vi "XYZ Joystick.vi"(0 "LSID":i32, 7 "Joystick on?":bool, 11 "error in (no error)":errorcluster) -> (15 "error out":errorcluster)   [LabVIEW 2014]
uses:
  <userlib>/Tango_DLL/Tango_DLL.lvlib
panel:
  # "LICENSED MATERIALS – PROPERTY OF IBM\nCopyright IBM Corp. 2016,\nALL RIGHTS RESERVED"
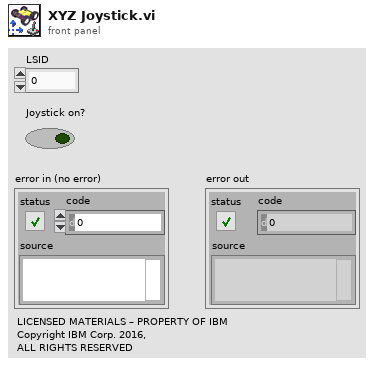
[diagram p1: front panel]
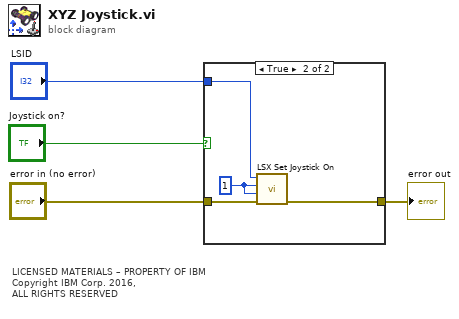
[diagram p0: block diagram]
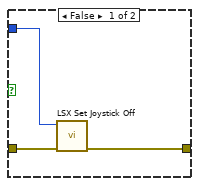
[diagram p2: hidden frame]
diagram:
  # "LICENSED MATERIALS – PROPERTY OF IBM\nCopyright IBM Corp. 2016,\nALL RIGHTS RESERVED"
  n1 = case shown="True" "Joystick on?" {
    tunnel: "error in (no error)" -> [w7 w11]
    tunnel: [w6 w10] -> w2
    tunnel: "LSID" -> [w5 w9]
    frame False {
      n2 = call <userlib>:"LSX Set Joystick Off.vi"("error in (no error)"=w7, "lLSID"=w5) -> ("error out"=w6:errorcluster)  [unwired: 8 in, 1 out]
    }
    frame True {
      w8 = 1 ("bPositionCount")
      n3 = call <userlib>:"LSX Set Joystick On.vi"("error in (no error)"=w11, "bEncoder"=w8, "bPositionCount"=w8, "lLSID"=w9) -> ("error out"=w10:errorcluster)  [unwired: 6 in, 1 out]
    }
  }
  "error out" <- w2
